vi "Configure Measurement.vi"(8 "error in (no error)":errorcluster, 10 "Params":variant, 11 "NI DMM in":refnum<class "NI DMM.lvclass">) -> (0 "error out":errorcluster, 3 "NI DMM out":refnum<class "NI DMM.lvclass">)   [LabVIEW 2020, in "NI DMM.lvlib" / "NI DMM.lvclass"]
uses:
  NI DMM.lvclass
  <instrlib>/niDMM/nidmm.llb/niDMM Function.ctl
  NI DMM.lvclass/NI DMM.ctl
  <instrlib>/niDMM/nidmm.llb/niDMM Configure Measurement Digits.vi
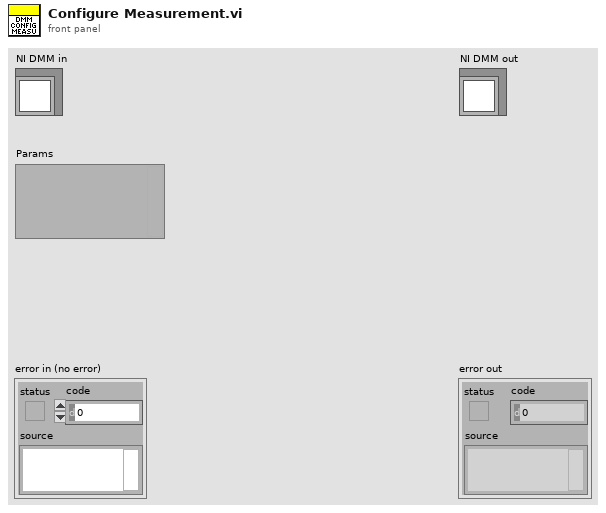
[diagram p1: front panel]
types:
  T1 = typedef "niDMM Function.ctl" = enum16{"DC Volts", "AC Volts", "DC Current", "AC Current", "2-wire Resistance", "4-wire Resistance", "Diode", "Frequency", "Period", "AC Volts DC Coupled", "Capacitance", "Inductance", "Temperature"}
  T2 = cluster{"Function":T1, "Resolution":dbl, "Range":dbl}
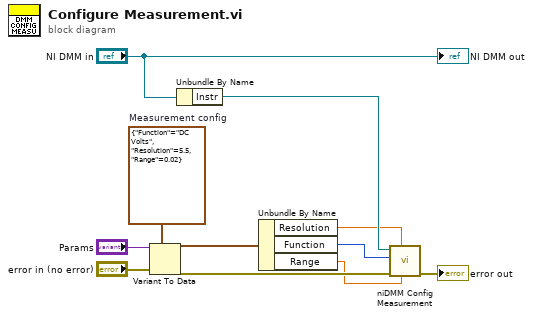
[diagram p0: block diagram]
diagram:
  w7 = T2 {"Function"=enum."DC Volts", "Resolution"=5.5, "Range"=0.02}  # Measurement config
  n1 = Variant To Data(error in="error in (no error)", type=w7, Variant="Params") -> (data=w5:T2, error out=w6:errorcluster)
  n2 = Unbundle By Name("NI DMM in") -> ("Instr"=w10:refnum<k15>)
  n3 = Unbundle By Name(w5) -> ("Resolution"=w3:dbl, "Function"=w4:T1, "Range"=w2:dbl)
  n4 = call-poly <instrlib>:"niDMM Config Measurement.vi"("Range"=w2, "Resolution in Digits"=w3, "error in (no error)"=w6, "Function"=w4, "instrument handle"=w10) -> ("error out"=→"error out":errorcluster)  [unwired: 5 in, 1 out]
  "NI DMM out" <- "NI DMM in"
